vi "Set_Bandwidth_DHPVA-100.vi"(3 "error in":errorcluster, 4 "Status":i32, 5 "Bandwidth":enum16{"10 MHz", "100 MHz"}(ring), 6 "index":i32) -> (0 "error out":errorcluster, 1 "Status_out":i32, 2 "index_out":i32)   [LabVIEW 2010, in "FEMTO_LUCI-10.lvlib"]
doc: "This functions sets the bandwidth of the selected device."
uses:
  <userlib>/FEMTO/FEMTO_LUCI-10.lvlib
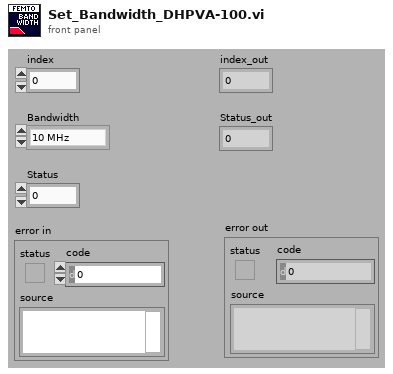
[diagram p1: front panel]
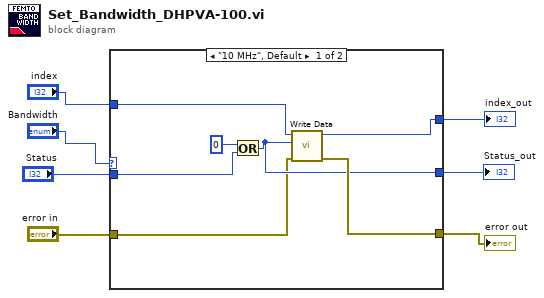
[diagram p0: block diagram]
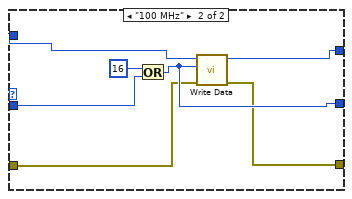
[diagram p2: hidden frame]
diagram:
  n1 = case shown="\"10 MHz\", Default" "Bandwidth" {
    tunnel: [w10 w21] -> w7
    tunnel: "Status" -> [w8 w20]
    tunnel: [w11 w19] -> w5
    tunnel: "error in" -> [w9 w18]
    tunnel: [w12 w17] -> w3
    tunnel: "index" -> [w13 w16]
    frame "10 MHz", Default {
      n2 = Or(x=0 ("data_low"), y=w8) -> (x .or. y?=w10:i32)
      n3 = call <userlib>:"Write Data.vi"("error in (no error)"=w9, "data_low"=w10, "index"=w13) -> ("error out"=w11:errorcluster, "index_out"=w12:i32)  [unwired: 1 in, 6 out]
    }
    frame "100 MHz" {
      n4 = Or(x=16 ("data_low"), y=w20) -> (x .or. y?=w21:i32)
      n5 = call <userlib>:"Write Data.vi"("error in (no error)"=w18, "data_low"=w21, "index"=w16) -> ("error out"=w19:errorcluster, "index_out"=w17:i32)  [unwired: 1 in, 6 out]
    }
  }
  "index_out" <- w3
  "error out" <- w5
  "Status_out" <- w7
